vi "Table Clear Selection.vi"(8 "error in":errorcluster, 11 "Table Ref In":refnum<vi>) -> (0 "error out":errorcluster, 3 "Table Ref Out":refnum<vi>)   [LabVIEW 2024]
uses:
  <vilib>/Utility/miscctls.llb/LVRowAndColumnTypeDef.ctl
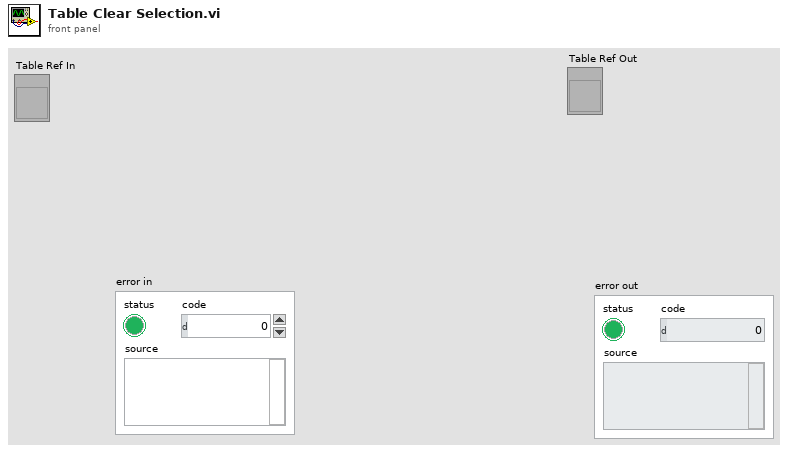
[diagram p1: front panel]
types:
  T1 = typedef "LVRowAndColumnTypeDef.ctl" = cluster{"Row":i32, "Column":i32}
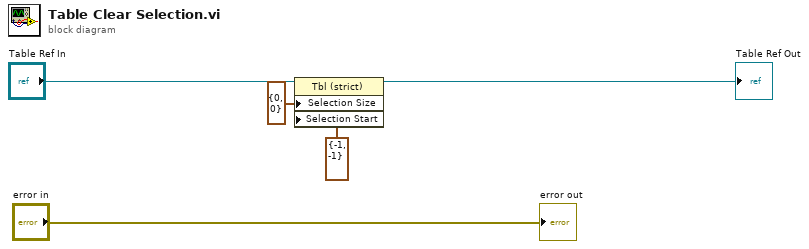
[diagram p0: block diagram]
diagram:
  n1 = property class="Tbl (strict)"(reference="Table Ref In", "Selection Size"=T1 {"Row"=0, "Column"=0}, "Selection Start"=T1 {"Row"=-1, "Column"=-1}) -> (reference out=→"Table Ref Out":refnum<vi>)  [unwired: 1 in, 1 out]
  "error out" <- "error in"
